vi "KinematicSlidingMode.vi"(3 "real v and w":cluster{"vr":dbl, "wr":dbl}, 4 "vck-1 wck-1":cluster{"vck-1":dbl, "wck-1":dbl}, 8 "error":cluster{"xe":dbl, "ye":dbl, "thetae":dbl}, 9 "vd and wd":T1, 10 "k":cluster{" k0":dbl, "k1":dbl, "k2":dbl}, 11 "P and Q":cluster{"P1":dbl, "P2":dbl, "Q1":dbl, "Q2":dbl}) -> (0 "vck wck":cluster{"vck":dbl, "wck":dbl}, 1 "w_L":dbl, 2 "w_R":dbl, 5 "ve we":cluster{"ve":dbl, "we":dbl})   [LabVIEW 2016]
panel:
  in  "l":dbl=0.365
  in  "r":dbl=0.046
  in  "deltat":dbl=0.15
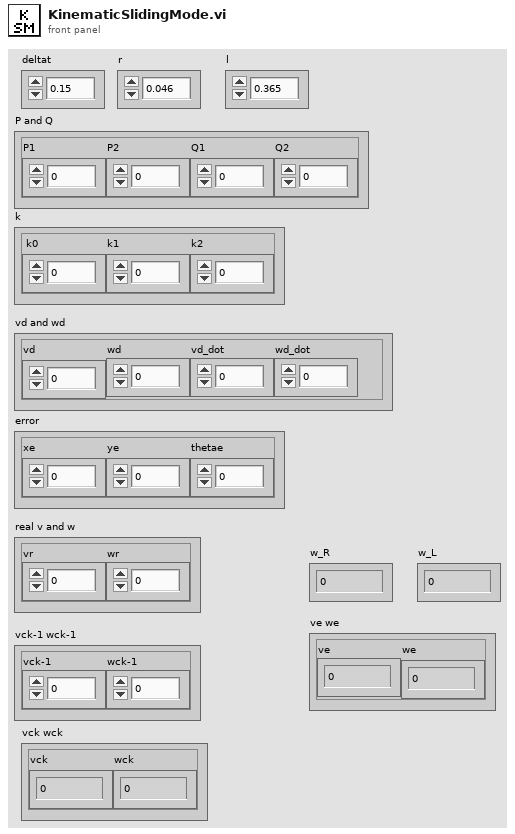
[diagram p1: front panel]
types:
  T1 = cluster{"vd":dbl, "wd":dbl, "vd_dot":dbl, "wd_dot":dbl}
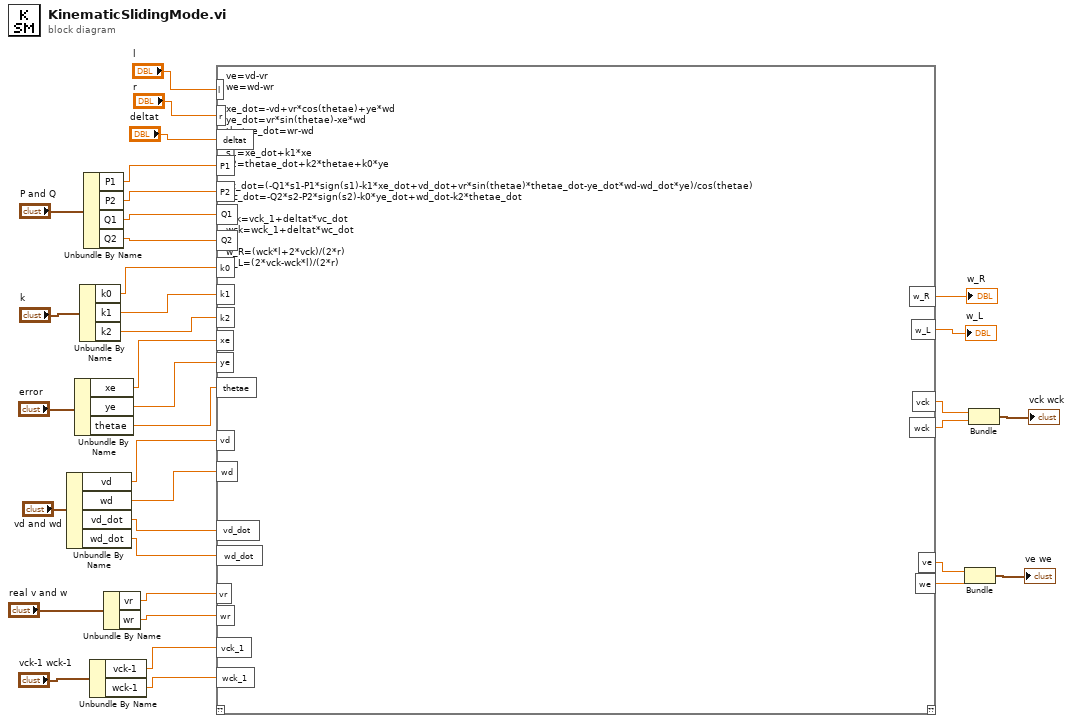
[diagram p0: block diagram]
diagram:
  n1 = Unbundle By Name("vd and wd") -> ("vd"=w18:dbl, "wd"=w17:dbl, "vd_dot"=w16:dbl, "wd_dot"=w15:dbl)
  n2 = Unbundle By Name("error") -> ("xe"=w22:dbl, "ye"=w21:dbl, "thetae"=w20:dbl)
  n3 = Unbundle By Name("k") -> ("k0"=w26:dbl, "k1"=w25:dbl, "k2"=w24:dbl)
  n4 = Unbundle By Name("P and Q") -> ("P1"=w31:dbl, "P2"=w30:dbl, "Q1"=w29:dbl, "Q2"=w28:dbl)
  n5 = Unbundle By Name("vck-1 wck-1") -> ("vck-1"=w8:dbl, "wck-1"=w7:dbl)
  n6 = Unbundle By Name("real v and w") -> ("vr"=w13:dbl, "wr"=w12:dbl)
  n7 = script code="ve=vd-vr\nwe=wd-wr\n\nxe_dot=-vd+vr*cos(thetae)+ye*wd\nye_dot=vr*sin(thetae)-xe*wd\nthetae_dot=wr-wd\n\ns1=xe_dot+k1*xe\ns2=thetae_dot+k2*thetae+k0*ye\n\nvc_dot=(-Q1*s1-P1*sign(s1)-k1*xe_dot+vd_dot+vr*sin(thetae)*thetae_dot-ye_dot*wd-wd_dot*ye)/cos(thetae)\nwc_dot=-Q2*s2-P2*sign(s2)-k0*ye_dot+wd_dot-k2*thetae_dot\n\nvck=vck_1+deltat*vc_dot\nwck=wck_1+deltat*wc_dot\n\nw_R=(wck*l+2*vck)/(2*r)\nw_L=(2*vck-wck*l)/(2*r)"("P1"=w31, "P2"=w30, "Q1"=w29, "Q2"=w28, "k0"=w26, "k1"=w25, "k2"=w24, "xe"=w22, "ye"=w21, "thetae"=w20, "vd"=w18, "wd"=w17, "deltat"="deltat", "vd_dot"=w16, "wd_dot"=w15, "vr"=w13, "wr"=w12, "vck_1"=w8, "wck_1"=w7, "l"="l", "r"="r") -> ("w_R"=→"w_R":dbl, "w_L"=→"w_L":dbl, "vck"=w6:dbl, "wck"=w5:dbl, "ve"=w2:dbl, "we"=w1:dbl)  [unwired: 1 in, 1 out]
  n8 = Bundle(w2, w1) -> (→"ve we":cluster{dbl, dbl})  [unwired: 1 in]
  n9 = Bundle(w6, w5) -> (→"vck wck":cluster{dbl, dbl})  [unwired: 1 in]
